vi "Find_Individual_Elements.vi"(7 "Array In":string[](array[string])) -> (8 "Array Out":string[](array[string]))   [LabVIEW 2012]
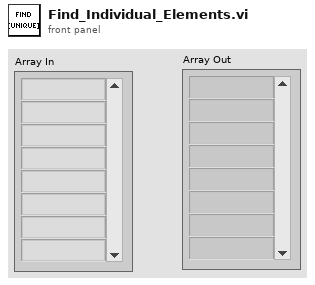
[diagram p1: front panel]
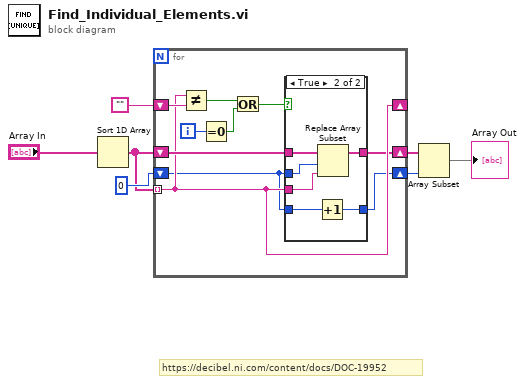
[diagram p0: block diagram]
diagram:
  # "https://decibel.ni.com/content/docs/DOC-19952"
  n1 = Sort 1D Array(array="Array In") -> (sorted array=w6:string[])
  n2 = for {
    shift-right: [w12] -> w5
    shift-left: w6 -> [w16]
    shift-right: [w13] -> w4
    shift-left: 0 -> [w14]
    tunnel: w6 -> [w15] mode=indexing
    shift-right: [w15] -> _
    shift-left: "" -> [w17]
    i -> [w11]
    n3 = Not Equal?(x=w15, y=w17) -> (x != y?=w10:bool)
    n4 = Equal To 0?(x=w11) -> (x = 0?=w9:bool)
    n5 = Or(x=w10, y=w9) -> (x .or. y?=w8:bool)
    n6 = case shown="True" w8 {
      tunnel: w16 -> [w19 w25]
      tunnel: w14 -> [_ w24]
      tunnel: w15 -> [_ w23]
      tunnel: w14 -> [w18 w22]
      tunnel: [w18 w21] -> w13
      tunnel: [w19 w20] -> w12
      frame False {
      }
      frame True {
        n7 = Increment(x=w22) -> (x+1=w21:i32)
        n8 = Replace Array Subset(array=w25, new element=w23, index=w24) -> (w20:string[])
      }
    }
  }
  n9 = Array Subset(array=w5, length=w4) -> (→"Array Out":string[])  [unwired: 1 in]
